vi "Get Date & Time_TV.vi"() -> (0 "Time":string, 3 "Date":string)   [LabVIEW 2020]
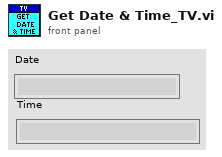
[diagram p1: front panel]
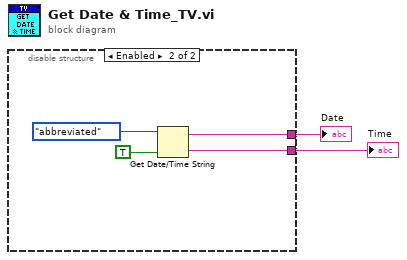
[diagram p0: block diagram]
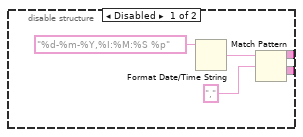
[diagram p2: hidden frame]
diagram:
  n1 = disable-structure shown="Enabled" {
    disable-tunnel: [w4 w8] -> w2
    disable-tunnel: [w3 w9] -> w1
    frame Disabled {
      n2 = Format Date/Time String(time format string (%c)="%d-%m-%Y,%I:%M:%S %p") -> (date/time string=w6:string)  [unwired: 2 out]
      n3 = Match Pattern(string=w6, regular expression=",") -> (before substring=w3:string, after substring=w4:string)  [unwired: 3 out]
    }
    frame Enabled {
      n4 = Get Date/Time String(date format (0)=enum16{"short", "long", "abbreviated"}."abbreviated", want seconds? (F)=TRUE) -> (date string=w9:string, time string=w8:string)  [unwired: 1 out]
    }
  }
  "Date" <- w1
  "Time" <- w2
